vi "VI Server Project.vi"() -> ()   [LabVIEW 2009]
panel:
  out "error out":errorcluster
  in  "port number or service name (3363)":u16=3363
  in  "machine name (\"\":  open local reference)":string="127.0.0.1"
  out "Version Number 2":u32=151027712 format="%.0x"
  out "Get VI Editor Version":string="9.0"
  in  "VI Path":path=path "C:/SVN/[E]-Engine/E0001/E0001.lvproj"
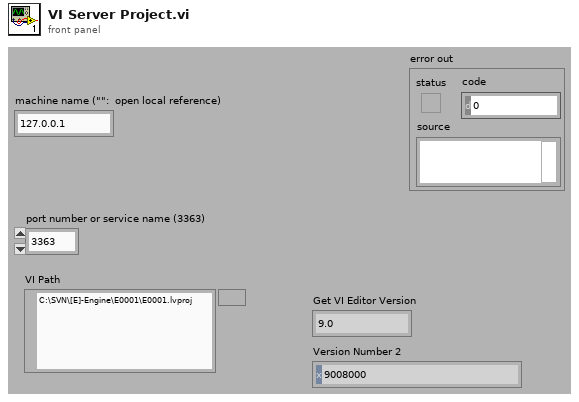
[diagram p1: front panel]
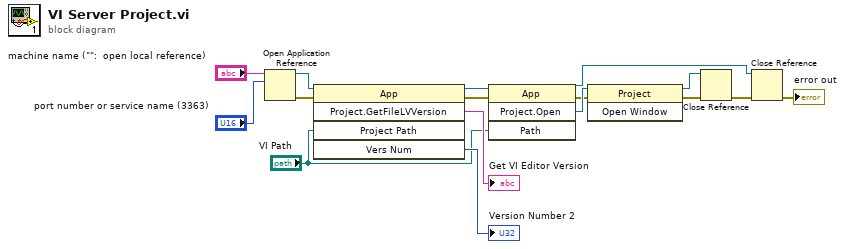
[diagram p0: block diagram]
diagram:
  n1 = Open Application Reference(10:"port number or service name (3363)", 11:"machine name (\"\":  open local reference)") -> (0:w10:errorcluster, 3:w11:refnum<vi>)  [unwired: 2 in]
  n2 = invoke class="App" method="Project.GetFileLVVersion"(reference=w11, error in=w10, "Project Path"="VI Path") -> (reference out=w9:refnum<vi>, error out=w5:errorcluster, "Project.GetFileLVVersion"=→"Get VI Editor Version":string, "Vers Num"=→"Version Number 2":u32)  [unwired: 2 in, 1 out]
  n3 = invoke class="App" method="Project.Open"(reference=w9, error in=w5, "Path"="VI Path") -> (reference out=w7:refnum<vi>, error out=w4:errorcluster, "Project:Open"=w8:refnum<vi>)  [unwired: 1 in, 1 out]
  n4 = invoke class="Project" method="Open Window"(reference=w8, error in=w4) -> (reference out=w6:refnum<vi>, error out=w3:errorcluster)  [unwired: 1 in, 1 out]
  n5 = Close Reference(reference=w6, error in (no error)=w3) -> (error out=w2:errorcluster)
  n6 = Close Reference(reference=w7, error in (no error)=w2) -> (error out=→"error out":errorcluster)
